vi "CAN_Init.vi"(0 "设备类型":u16(ring)=4 items=["PCI5121"=1, "PCI9810"=2, "USBCAN1"=3, "USBCAN2"=4, "PCI9820"=5, "CAN232"=6, "PCI5110"=7, "CANLite(mini)"=8, "ISA9620"=9, "ISA5420"=10, "PC104CAN"=11, "CANETE"=12, "DNP9810"=13], 1 "设备索引":u16(ring) items=["0", "1", "2", "3", "4", "5", "6", "7", "8", "9", "10", "11", "12", "13", "14", "15", ""], 2 "波特率":T2(ring)=enum."250Kbps", 3 "CAN路数":u16(ring) items=["0", "1"], 4 "操作类型":enum16{"初始化CAN", "关闭CAN"}(ring), 5 "error in (no error)":errorcluster caption="错误输入（无错误）", 6 "滤波方式":u8(ring)=1 items=["Dual Filter", "Single Filter"], 7 "Accept Code":u32 format="%08x", 10 "工作方式":u8(ring) items=["Normal", "Listen Only"], 11 "Mask Code":u32=4294967295 format="%08x") -> (14 "CAN 操作结果":bool=TRUE, 19 "error out":errorcluster caption="错误输出")   [LabVIEW 2013]
uses:
  data/ControlCAN.dll
panel:
  in  "VCI_INIT_CONFIG":T1={"AccCode"=0, "AccMask"=4294967295, "Reserved"=0, "Filter"=0, "Timing0"=191, "Timing1"=255, "Mode"=0}
  in  "DeviceType 5":u16(ring)=1 items=["PCI5121"=1, "PCI9810"=2, "USBCAN1"=3, "USBCAN2"=4, "PCI9820"=5, "CAN232"=6, "PCI5110"=7, "CANLite(mini)"=8, "ISA9620"=9, "ISA5420"=10, "PC104CAN"=11, "CANETE"=12, "DNP9810"=13]
  in  "CAN Channel 3":u16(ring) items=["0", "1"]
  in  "DeviceType 4":u16(ring)=1 items=["PCI5121"=1, "PCI9810"=2, "USBCAN1"=3, "USBCAN2"=4, "PCI9820"=5, "CAN232"=6, "PCI5110"=7, "CANLite(mini)"=8, "ISA9620"=9, "ISA5420"=10, "PC104CAN"=11, "CANETE"=12, "DNP9810"=13]
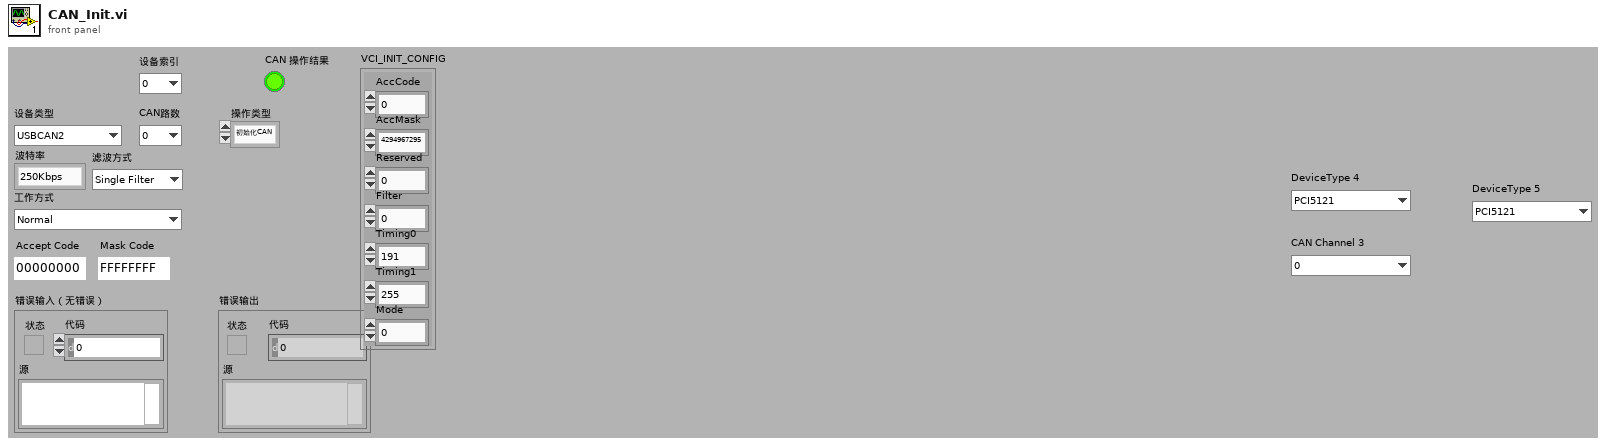
[diagram p1: front panel]
types:
  T1 = cluster{"AccCode":u32, "AccMask":u32, "Reserved":u32, "Filter":u8, "Timing0":u8, "Timing1":u8, "Mode":u8}
  T2 = enum16{"5Kbps", "10Kbps", "20Kbps", "40Kbps", "50Kbps", "80Kbps", "100Kbps", "125Kbps", "200Kbps", "250Kbps", "400Kbps", "500Kbps", "666Kbps", "800Kbps", "1000Kbps"}
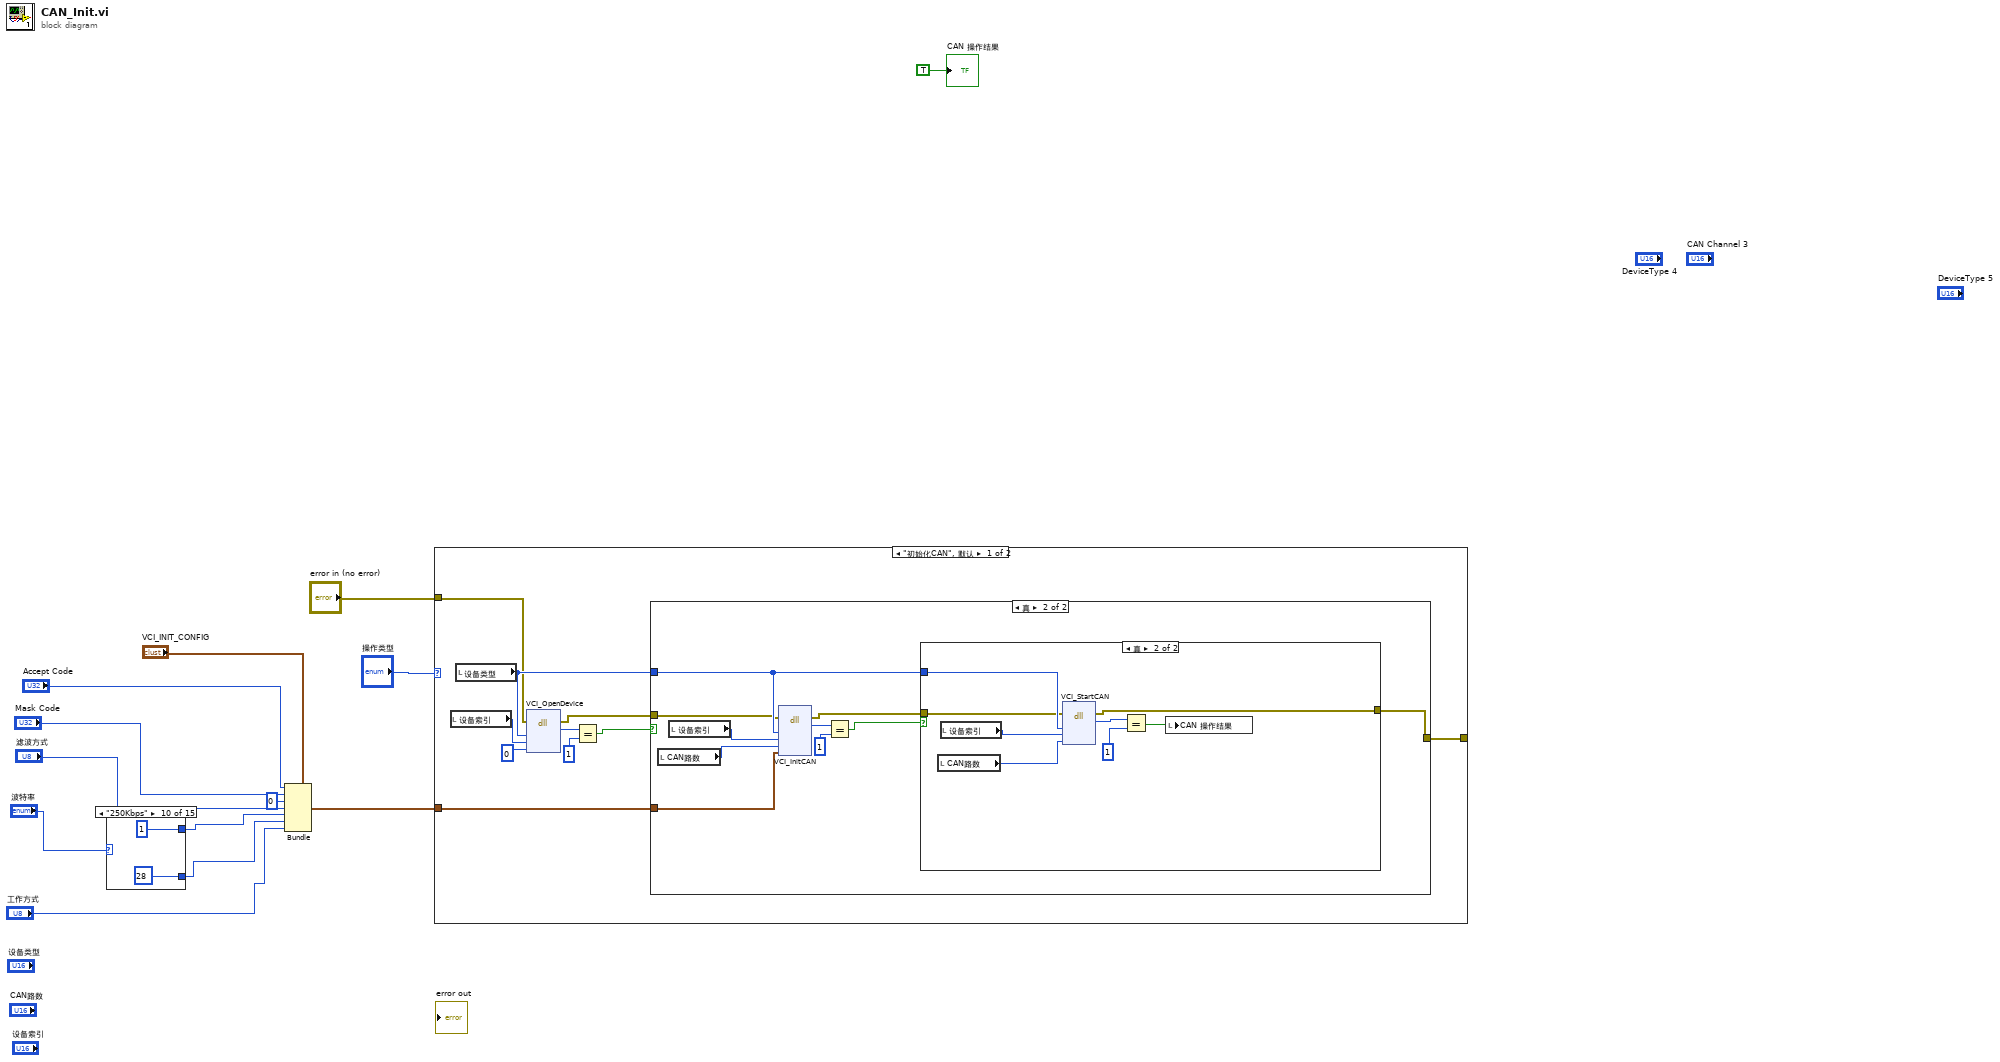
[diagram p0: block diagram]
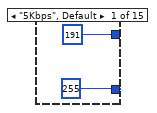
[diagram p2: hidden frame]
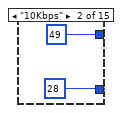
[diagram p3: hidden frame]
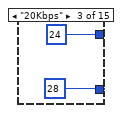
[diagram p4: hidden frame]
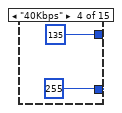
[diagram p5: hidden frame]
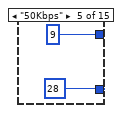
[diagram p6: hidden frame]
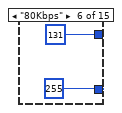
[diagram p7: hidden frame]
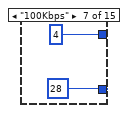
[diagram p8: hidden frame]
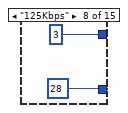
[diagram p9: hidden frame]
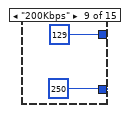
[diagram p10: hidden frame]
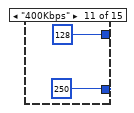
[diagram p11: hidden frame]
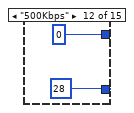
[diagram p12: hidden frame]
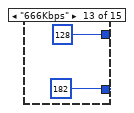
[diagram p13: hidden frame]
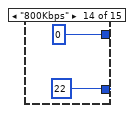
[diagram p14: hidden frame]
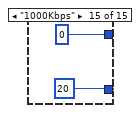
[diagram p15: hidden frame]
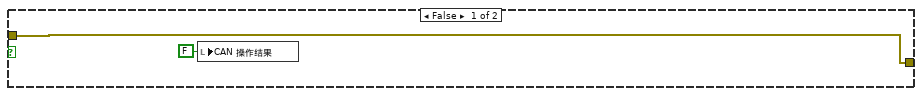
[diagram p16: hidden frame]
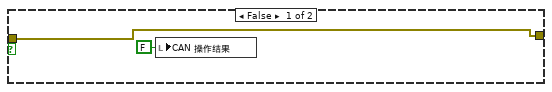
[diagram p17: hidden frame]
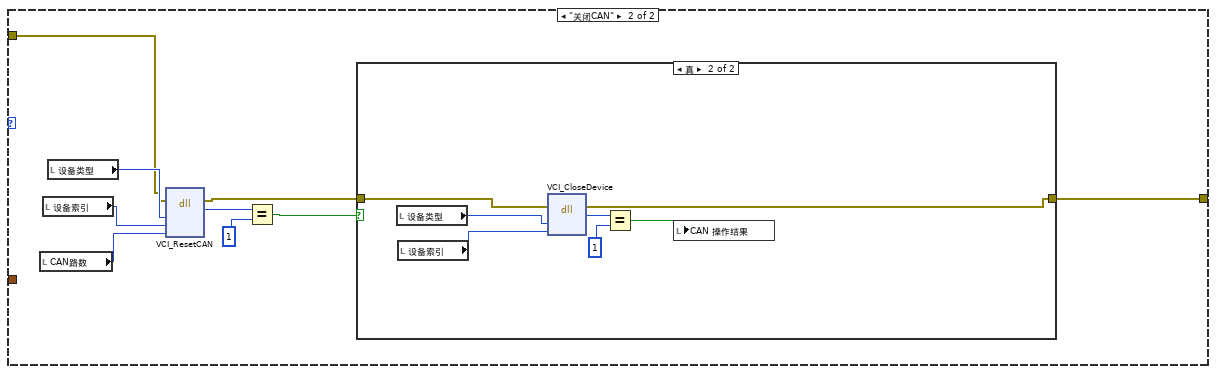
[diagram p18: hidden frame]
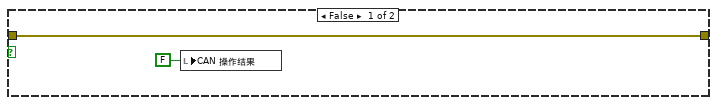
[diagram p19: hidden frame]
diagram:
  n1 = case shown="\"250Kbps\"" "波特率" {
    tunnel: [191 49 24 135 9 131 4 3 129 1 128 0 128 0 0] -> w12
    tunnel: [255 28 28 255 28 255 28 28 250 28 250 28 182 22 20] -> w11
    frame "5Kbps", Default {
    }
    frame "10Kbps" {
    }
    frame "20Kbps" {
    }
    frame "40Kbps" {
    }
    frame "50Kbps" {
    }
    frame "80Kbps" {
    }
    frame "100Kbps" {
    }
    frame "125Kbps" {
    }
    frame "200Kbps" {
    }
    frame "250Kbps" {
    }
    frame "400Kbps" {
    }
    frame "500Kbps" {
    }
    frame "666Kbps" {
    }
    frame "800Kbps" {
    }
    frame "1000Kbps" {
    }
  }
  n2 = Bundle(cluster="VCI_INIT_CONFIG", "AccCode"="Accept Code", "AccMask"="Mask Code", "Reserved"=u32 0, "Filter"="滤波方式", "Timing0"=w12, "Timing1"=w11, "Mode"="工作方式") -> (w7:T1)
  n3 = case shown="\"初始化CAN\", 默认" "操作类型" {
    tunnel: w7 -> [w47 _]
    tunnel: "error in (no error)" -> [w46 w78]
    tunnel: [w44 w76] -> _
    frame "初始化CAN", Default {
      n4 = local read "设备索引"() -> (w50:u16)
      n5 = local read "设备类型"() -> (w48:u16)
      n6 = dll-call lib="PTH1Yabs FBluewave New Energy\t上位机BMS_Monitor - 91版 新源dataControlCAN.dll" fn="VCI_OpenDevice"(error in=w46, "DevType"=w48, "DevIndex"=w50, "Reserved"=0) -> (error out=w45:errorcluster, "返回类型"=w52:u32)  [unwired: 3 in, 3 out]
      n7 = Equal?(x=w52, y=u32 1) -> (x = y?=w49:bool)
      n8 = case shown="真" w49 {
        tunnel: w48 -> [_ w60]
        tunnel: w47 -> [_ w59]
        tunnel: w45 -> [w54 w58]
        tunnel: [w54 w56] -> w44
        frame False {
          n9 = local write "CAN 操作结果"(FALSE ("初始化结果")) -> ()
        }
        frame True {
          n10 = local read "CAN路数"() -> (w62:u16)
          n11 = local read "设备索引"() -> (w63:u16)
          n12 = dll-call lib="PTH1Yabs FBluewave New Energy\t上位机BMS_Monitor - 91版 新源dataControlCAN.dll" fn="VCI_InitCAN"(error in=w58, "DeviceType"=w60, "DeviceInd"=w63, "CANInd"=w62, "VCI_INIT_CONFIG"=w59) -> (error out=w57:errorcluster, w64:u32)  [unwired: 3 in, 4 out]
          n13 = Equal?(x=w64, y=u32 1) -> (x = y?=w61:bool)
          n14 = case shown="真" w61 {
            tunnel: w60 -> [_ w73]
            tunnel: w57 -> [w66 w69]
            tunnel: [w66 w68] -> w56
            frame False {
              n15 = local write "CAN 操作结果"(FALSE ("初始化结果")) -> ()
            }
            frame True {
              n16 = local read "CAN路数"() -> (w71:u16)
              n17 = local read "设备索引"() -> (w72:u16)
              n18 = dll-call lib="PTH1Yabs FBluewave New Energy\t上位机BMS_Monitor - 91版 新源dataControlCAN.dll" fn="VCI_StartCAN"(error in=w69, "DeviceType"=w73, "DeviceInd"=w72, "CANInd"=w71) -> (error out=w68:errorcluster, "返回类型"=w74:u32)  [unwired: 2 in, 4 out]
              n19 = Equal?(x=w74, y=u32 1) -> (x = y?=w70:bool)
              n20 = local write "CAN 操作结果"(w70) -> ()
            }
          }
        }
      }
    }
    frame "关闭CAN" {
      n21 = local read "CAN路数"() -> (w79:u16)
      n22 = local read "设备索引"() -> (w80:u16)
      n23 = local read "设备类型"() -> (w81:u16)
      n24 = dll-call lib="PTH1Yabs FBluewave New Energy\t上位机BMS_Monitor - 91版 新源dataControlCAN.dll" fn="VCI_ResetCAN"(error in=w78, "DeviceType"=w81, "DeviceInd"=w80, "CANInd"=w79) -> (error out=w77:errorcluster, "返回类型"=w83:u32)  [unwired: 2 in, 4 out]
      n25 = Equal?(x=w83, y=u32 1) -> (x = y?=w82:bool)
      n26 = case shown="真" w82 {
        tunnel: w77 -> [w85 w88]
        tunnel: [w85 w87] -> w76
        frame False {
          n27 = local write "CAN 操作结果"(FALSE ("CAN 操作结果")) -> ()
        }
        frame True {
          n28 = local read "设备类型"() -> (w91:u16)
          n29 = local read "设备索引"() -> (w90:u16)
          n30 = dll-call lib="PTH1Yabs FBluewave New Energy\t上位机BMS_Monitor - 91版 新源dataControlCAN.dll" fn="VCI_CloseDevice"(error in=w88, "DeviceType"=w91, "DeviceInd"=w90) -> (error out=w87:errorcluster, w92:u32)  [unwired: 2 in, 3 out]
          n31 = Equal?(x=w92, y=u32 1) -> (x = y?=w89:bool)
          n32 = local write "CAN 操作结果"(w89) -> ()
        }
      }
    }
  }
  "CAN 操作结果" <- TRUE ("CAN 操作结果")
